vi "Write VS output FIFO.vi"(8 "error in (no error)":errorcluster, 10 "CD  state in":T1[](array[typedef]), 11 "Refnum in":refnum<k33>) -> (0 "error out":errorcluster, 2 "CD State out":T1[](array[typedef]))   [LabVIEW 2014, in "UEGO Sim Engine.lvlib"]
uses:
  UEGO Sim Engine.lvlib
  UEGO CD state.ctl
  Shared/UEGO fpga inputs.ctl
  Shared/UEGO fpga outputs.ctl
  Shared/VS input channels.ctl
  Shared/VS output channels.ctl
  Shared/UEGO Sim Shared.lvlib
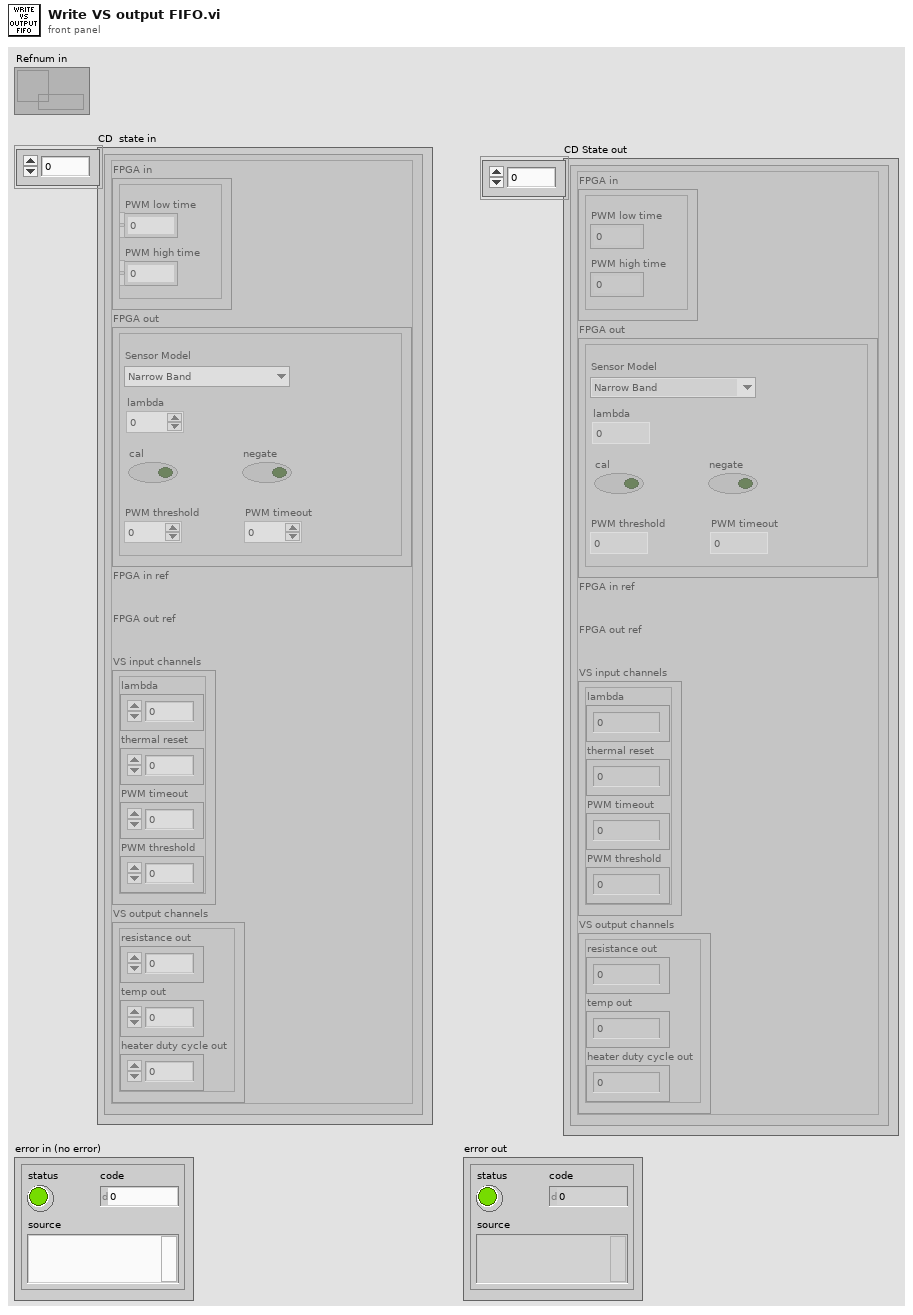
[diagram p1: front panel]
types:
  T1 = typedef "UEGO Sim Engine.lvlib/UEGO CD state.ctl" = cluster{"FPGA in":T2, "FPGA out":T3, "FPGA in ref":refnum<k20>, "FPGA out ref":refnum<k20>, "VS input channels":T5, "VS output channels":T6}
  T2 = typedef "UEGO Sim Shared.lvlib/UEGO fpga inputs.ctl" = cluster{"PWM low time":u32, "PWM high time":u32}
  T3 = typedef "UEGO Sim Shared.lvlib/UEGO fpga outputs.ctl" = cluster{"Sensor Model":T4, "lambda":fxp<+,12,3>, "cal":bool, "negate":bool, "PWM threshold":i16, "PWM timeout":u32}
  T4 = typedef "UEGO Sim Shared.lvlib/sensor models" = enum16{"Narrow Band", "Bosch 4.2", "Bosch 4.9"}
  T5 = typedef "UEGO Sim Shared.lvlib/VS input channels.ctl" = cluster{"lambda":dbl, "thermal reset":dbl, "PWM timeout":dbl, "PWM threshold":dbl}
  T6 = typedef "UEGO Sim Shared.lvlib/VS output channels.ctl" = cluster{"resistance out":dbl, "temp out":dbl, "heater duty cycle out":dbl}
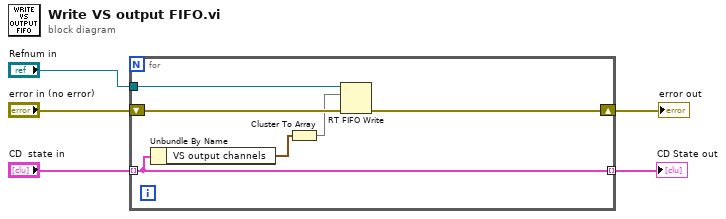
[diagram p0: block diagram]
diagram:
  n1 = for {
    tunnel: "Refnum in" -> [w11]
    tunnel: "CD  state in" -> [w6] mode=indexing
    tunnel: [w6] -> w1 mode=indexing
    shift-right: [w10] -> w3
    shift-left: "error in (no error)" -> [w9]
    n2 = Unbundle By Name(w6) -> ("VS output channels"=w8:T6)
    n3 = Cluster To Array(cluster=w8) -> (array=w7:dbl[])
    n4 = RT FIFO Write(0:w11, 1:w7, 3:w9) -> (11:w10:errorcluster)  [unwired: 1 in, 4 out]
  }
  "error out" <- w3
  "CD State out" <- w1
